vi "calibrate2.vi"(4 "stepAmp":i32, 5 "axis":i32, 6 "error_in":errorcluster, 7 "referenceIn":refnum<k24>) -> (0 "nForwardSteps":i32, 1 "nReverseSteps":i32, 2 "errorOut":errorcluster, 3 "referenceOut":refnum<k24>)   [LabVIEW 2020]
uses:
  C:/Program Files/Newport/Piezo Motion Control/Newport AG-UC2-UC8 Applet/Samples/LabVIEW 2009/AgilisCmdLib.dll
  Program Files/Newport/Piezo Motion Control/Newport AG-UC2-UC8 Applet/Samples/LabVIEW 2009/AgilisCmdLib.dll
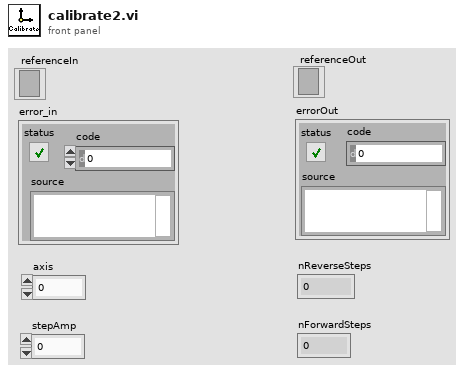
[diagram p1: front panel]
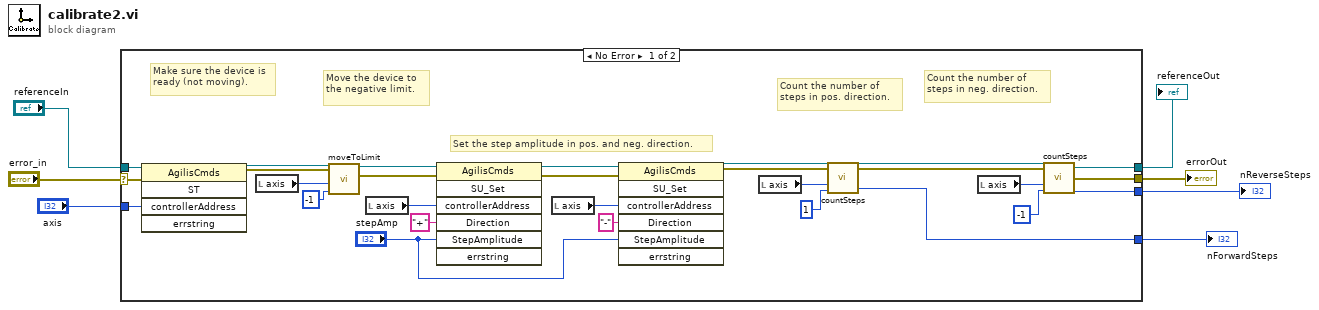
[diagram p0: block diagram]
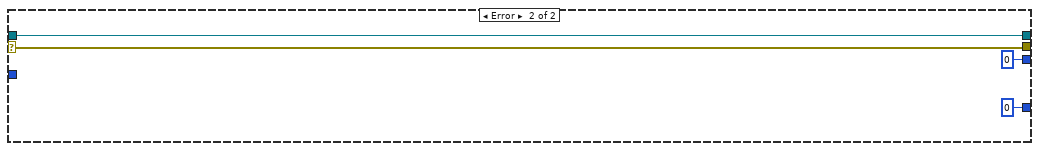
[diagram p2: hidden frame]
diagram:
  n1 = case shown="No Error" "error_in" {
    selector: "error_in" -> [w9 w38]
    tunnel: "referenceIn" -> [w35 w39]
    tunnel: "axis" -> [w34 _]
    tunnel: [w12 0 ("nSteps")] -> w5
    tunnel: [w11 w38] -> w4
    tunnel: [w10 w39] -> w3
    tunnel: [w8 0 ("nSteps")] -> w1
    frame No Error {
      # "Count the number of steps in neg. direction."
      # "Count the number of steps in pos. direction."
      # "Move the device to the negative limit."
      # "Set the step amplitude in pos. and neg. direction."
      # "Make sure the device is ready (not moving)."
      n2 = invoke class="AgilisCmds" method="ST"(reference=w35, error in=w9, "controllerAddress"=w34) -> (reference out=w33:refnum<k24>, error out=w32:errorcluster)  [unwired: 2 in, 3 out]
      n3 = local read "axis"() -> (w31:i32)
      n4 = call "moveToLimit.vi"("direction"=-1, "axis"=w31, "errorIn"=w32, "referenceIn"=w33) -> ("errorOut"=w28:errorcluster, "referenceOut"=w29:refnum<k24>)
      n5 = local read "axis"() -> (w27:i32)
      n6 = invoke class="AgilisCmds" method="SU_Set"(reference=w29, error in=w28, "controllerAddress"=w27, "Direction"="+", "StepAmplitude"="stepAmp") -> (reference out=w25:refnum<k24>, error out=w24:errorcluster)  [unwired: 2 in, 5 out]
      n7 = local read "axis"() -> (w23:i32)
      n8 = invoke class="AgilisCmds" method="SU_Set"(reference=w25, error in=w24, "controllerAddress"=w23, "Direction"="-", "StepAmplitude"="stepAmp") -> (reference out=w20:refnum<k24>, error out=w19:errorcluster)  [unwired: 2 in, 5 out]
      n9 = local read "axis"() -> (w18:i32)
      n10 = call "countSteps.vi"("direction"=1, "axis"=w18, "errorIn"=w19, "referenceIn"=w20) -> ("nSteps"=w8:i32, "error_out"=w15:errorcluster, "referenceOut"=w16:refnum<k24>)
      n11 = local read "axis"() -> (w14:i32)
      n12 = call "countSteps.vi"("direction"=-1, "axis"=w14, "errorIn"=w15, "referenceIn"=w16) -> ("nSteps"=w12:i32, "error_out"=w11:errorcluster, "referenceOut"=w10:refnum<k24>)
    }
    frame Error {
    }
  }
  "nReverseSteps" <- w5
  "errorOut" <- w4
  "referenceOut" <- w3
  "nForwardSteps" <- w1
